vi "GSIOC immediate.vi"(8 "error in (no error)":errorcluster, 10 "Immediate command":string, 11 "VISA resource name":refnum<visa-resource-name>="COM1") -> (0 "error out":errorcluster, 2 "Receive string":string, 3 "VISA resource name":refnum<visa-resource-name>="COM1")   [LabVIEW 2015]
panel:
  out "got char":bool
  out "loop":i32
  out "bytes at port":bool
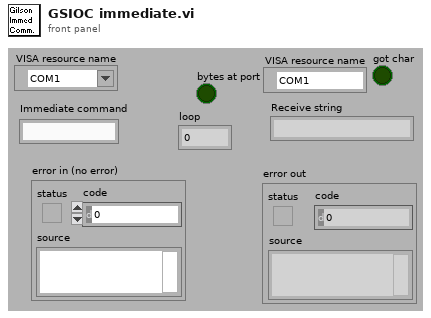
[diagram p1: front panel]
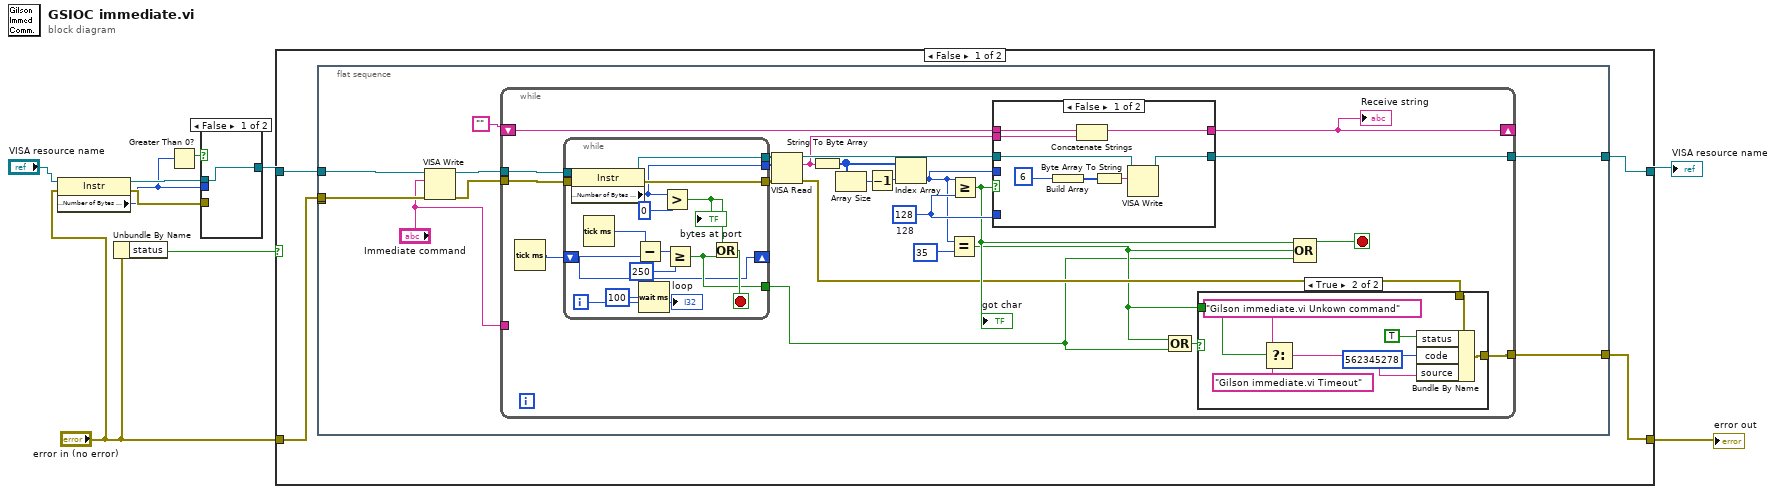
[diagram p0: block diagram]
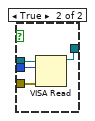
[diagram p2: hidden frame]
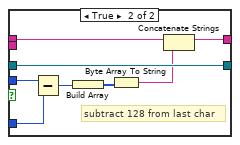
[diagram p4: hidden frame]
diagram:
  n1 = property class="Instr"(reference="VISA resource name", error in="error in (no error)") -> (reference out=w3:refnum<visa-resource-name>, error out=w4:errorcluster, "Serial Settings:Number of Bytes at Serial Port"=w2:u32)
  n2 = Unbundle By Name("error in (no error)") -> ("status"=w10:bool)
  n3 = Greater Than 0?(x=w2) -> (x > 0?=w1:bool)
  n4 = case shown="False" w1 {
    tunnel: [w11 w15] -> w6
    tunnel: w4 -> [_ w14]
    tunnel: w3 -> [w11 w13]
    tunnel: w2 -> [_ w12]
    frame False {
    }
    frame True {
      n5 = VISA Read(VISA resource name=w13, byte count=w12, error in (no error)=w14) -> (VISA resource name out=w15:refnum<visa-resource-name>)  [unwired: 3 out]
    }
  }
  n6 = case shown="False" w10 {
    tunnel: "error in (no error)" -> [w19 w93]
    tunnel: [w18 w93] -> w9
    tunnel: [w17 w92] -> w8
    tunnel: w6 -> [w16 w92]
    frame False {
      n7 = flat-sequence {
        tunnel: w16 -> [w27]
        tunnel: [w26] -> _
        tunnel: w19 -> [w26]
        tunnel: [w22] -> w18
        tunnel: [w21] -> w17
        frame #0 {
          n8 = VISA Write(VISA resource name=w27, write buffer="Immediate command", error in (no error)=w26) -> (VISA resource name out=w24:refnum<visa-resource-name>, error out=w25:errorcluster)  [unwired: 1 out]
          n9 = while {
            tunnel: w25 -> [w50]
            tunnel: w24 -> [w49]
            shift-right: [w33] -> _
            shift-left: "" -> [w46]
            tunnel: [w38] -> w22
            tunnel: [w34] -> w21
            tunnel: "Immediate command" -> [_]
            stop <- w41 stop-if-true
            w45 = u8 128  # 128
            n10 = Tick Count (ms)() -> (millisecond timer value=w35:u32)
            n11 = while {
              tunnel: [w75] -> w51
              tunnel: w50 -> [w74]
              tunnel: w49 -> [w73]
              tunnel: [w72] -> w48
              tunnel: [w68] -> w40
              tunnel: [w63] -> w32
              shift-right: [w62] -> _
              shift-left: w35 -> [w62]
              i -> [w61]
              stop <- w64 stop-if-true
              n12 = property class="Instr"(reference=w73, error in=w74) -> (reference out=w72:refnum<visa-resource-name>, error out=w75:errorcluster, "Serial Settings:Number of Bytes at Serial Port"=w68:u32)
              n13 = Tick Count (ms)() -> (millisecond timer value=w69:u32)
              n14 = Subtract(x=w69, y=w62) -> (x-y=w71:u32)
              n15 = Wait (ms)(milliseconds to wait=u32 100) -> ()  [unwired: 1 out]
              n16 = Greater?(x=w68, y=u32 0) -> (0:w65:bool)
              "bytes at port" <- w65
              n17 = Greater Or Equal?(x=w71, y=u32 250) -> (x >= y?=w63:bool)
              n18 = Or(x=w65, y=w63) -> (x .or. y?=w64:bool)
              "loop" <- w61
            }
            n19 = VISA Read(VISA resource name=w48, byte count=w40, error in (no error)=w51) -> (VISA resource name out=w47:refnum<visa-resource-name>, read buffer=w31:string, error out=w37:errorcluster)  [unwired: 1 out]
            n20 = String To Byte Array(string=w31) -> (unsigned byte array=w29:u8[])
            n21 = Array Size(array=w29) -> (size(s)=w30:i32)
            n22 = Decrement(x=w30) -> (x-1=w28:i32)
            n23 = Index Array(array=w29, index=w28) -> (element=w44:u8)
            n24 = Equal?(x=w44, y=u8 35) -> (x = y?=w36:bool)
            n25 = Greater Or Equal?(x=w44, y=w45) -> (x >= y?=w42:bool)
            "got char" <- w42
            n26 = case shown="False" w42 {
              tunnel: w47 -> [w83 w91]
              tunnel: [w79 w91] -> w34
              tunnel: w46 -> [w78 w90]
              tunnel: [w77 w89] -> w33
              tunnel: w31 -> [w76 _]
              tunnel: w44 -> [_ w88]
              tunnel: w45 -> [_ w87]
              frame False {
                n27 = Build Array(u8 6) -> (w80:u8[])
                n28 = Concatenate Strings(w78, w76) -> (w77:string)
                n29 = Byte Array To String(unsigned byte array=w80) -> (string=w81:string)
                n30 = VISA Write(VISA resource name=w83, write buffer=w81) -> (VISA resource name out=w79:refnum<visa-resource-name>)  [unwired: 1 in, 2 out]
              }
              frame True {
                # "subtract 128 from last char"
                n31 = Subtract(x=w88, y=w87) -> (x-y=w86:u8)
                n32 = Build Array(w86) -> (w85:u8[])
                n33 = Byte Array To String(unsigned byte array=w85) -> (string=w84:string)
                n34 = Concatenate Strings(w90, w84) -> (w89:string)
              }
            }
            "Receive string" <- w33
            n35 = Compound Arithmetic op=OR(w36, w32) -> (w39:bool)
            n36 = case shown="True" w39 {
              tunnel: [w52 w59] -> w38
              tunnel: w37 -> [w52 w60]
              tunnel: w36 -> [_ w54]
              frame False {
              }
              frame True {
                n37 = Select(t="Gilson immediate.vi Unkown command", s=w54, f="Gilson immediate.vi Timeout") -> (s? t:f=w55:string)
                n38 = Bundle By Name(cluster=w60, "status"=TRUE, "code"=562345278, "source"=w55) -> (w59:errorcluster)
              }
            }
            n39 = Compound Arithmetic op=OR(w42, w36, w32) -> (w41:bool)
          }
        }
      }
    }
    frame True {
    }
  }
  "error out" <- w9
  "VISA resource name" <- w8
